vi "读取服务器信息.vi"(8 "error in (no error)":errorcluster caption="错误输入（无错误）", 11 "TCP_client输入":refnum<class "TCP_client.lvclass">) -> (0 "error out":errorcluster caption="错误输出", 2 "服务器信息":cluster{"host":string, "port":u16}={"host"="121.36.219.111", "port"=10001}, 3 "TCP_client输出":refnum<class "TCP_client.lvclass">)   [LabVIEW 2022 SP3, in "update.lvlib" / "TCP_client.lvclass"]
uses:
  TCP_client.lvclass
  TCP_client.lvclass/TCP_client.ctl
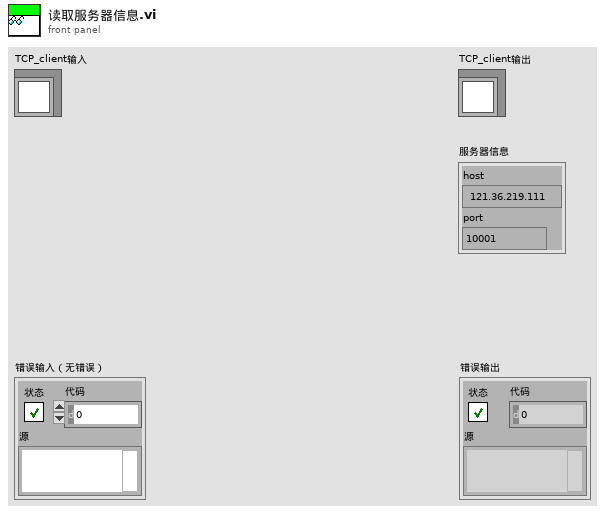
[diagram p1: front panel]
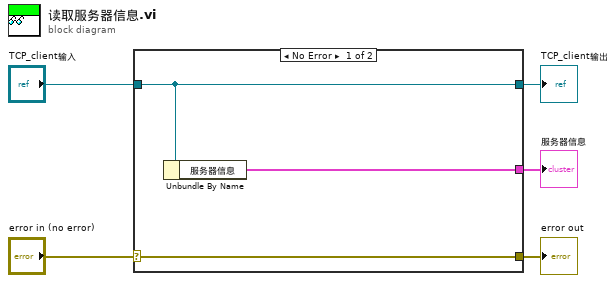
[diagram p0: block diagram]
diagram:
  n1 = case shown="No Error" "error in (no error)" {
    selector: "error in (no error)" -> [w8 w9]
    tunnel: [w8 w9] -> w4
    tunnel: [w7 w10] -> w2
    tunnel: "TCP_client输入" -> [w7 w10]
    tunnel: [w6 _] -> w1
    frame No Error {
      n2 = Unbundle By Name(w7) -> ("服务器信息"=w6:cluster{"host":string, "port":u16})
    }
    frame Error {
    }
  }
  "error out" <- w4
  "TCP_client输出" <- w2
  "服务器信息" <- w1
